vi "CameraSetup.vi"() -> ()   [LabVIEW 2015, in "CameraSetup.lvlib"]
uses:
  CameraSetup.lvlib
  <vilib>/userdefined/High Color/IMAQdx.ctl
  <vilib>/vision/driver/IMAQdx.llb/IMAQdx Acquisition Mode.ctl
  <vilib>/vision/driver/IMAQdx.llb/IMAQdx Buffer Number Mode.ctl
  <vilib>/vision/driver/NI_Vision_Acquisition_Software.lvlib
panel:
  in  "SaveConfig":bool caption="Save"
  in  "PageTab":T1(tab)
  in  "U32":u32(slide) min=720 max=720 step=1 scale=648.0..720.0
  in  "DBL":dbl(slide)=1e-06 min=0.0 max=3.999 step=1.0 scale=0.0..3.999
  in  "String":string
  in  "Ring":u32(ring) caption="Enum" items=["Bilinear", "VNG"]
  in  "Boolean":bool
  in  "Command":bool
  in  "Grab":bool
  out "Tooltip":string
  out "Image":T2(plugin-control)
  in  "Attribute":string(tree)
  in  "Cameras List":T3
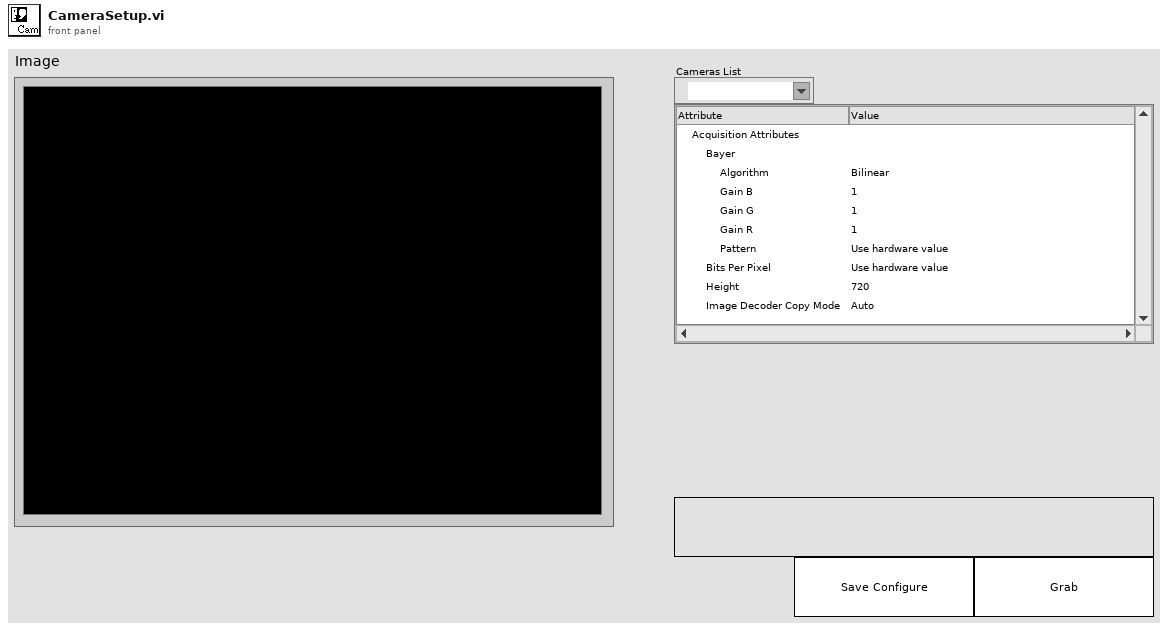
[diagram p1: front panel]
types:
  T1 = enum32{"U32", "DBL", "String", "Enum", "Bool", "Command"}
  T2 = typedef "IMAQ Image.ctl" = refnum<image>
  T3 = typedef "IMAQdx.ctl" = refnum<k21>
  T4 = cluster{"PageTab":refnum<vi>, "U32":refnum<vi>, "DBL":refnum<vi>, "String":refnum<vi>, "Enum":refnum<vi>, "Boolean":refnum<vi>, "Command":refnum<vi>}
  T5 = typedef "NI_Vision_Acquisition_Software.lvlib/IMAQdx Acquisition Mode.ctl" = enum32{"One Shot", "Continuous"}
  T6 = typedef "NI_Vision_Acquisition_Software.lvlib/IMAQdx Buffer Number Mode.ctl" = enum32{"Next", "Last", "Buffer Number", "Every", "Last New"}
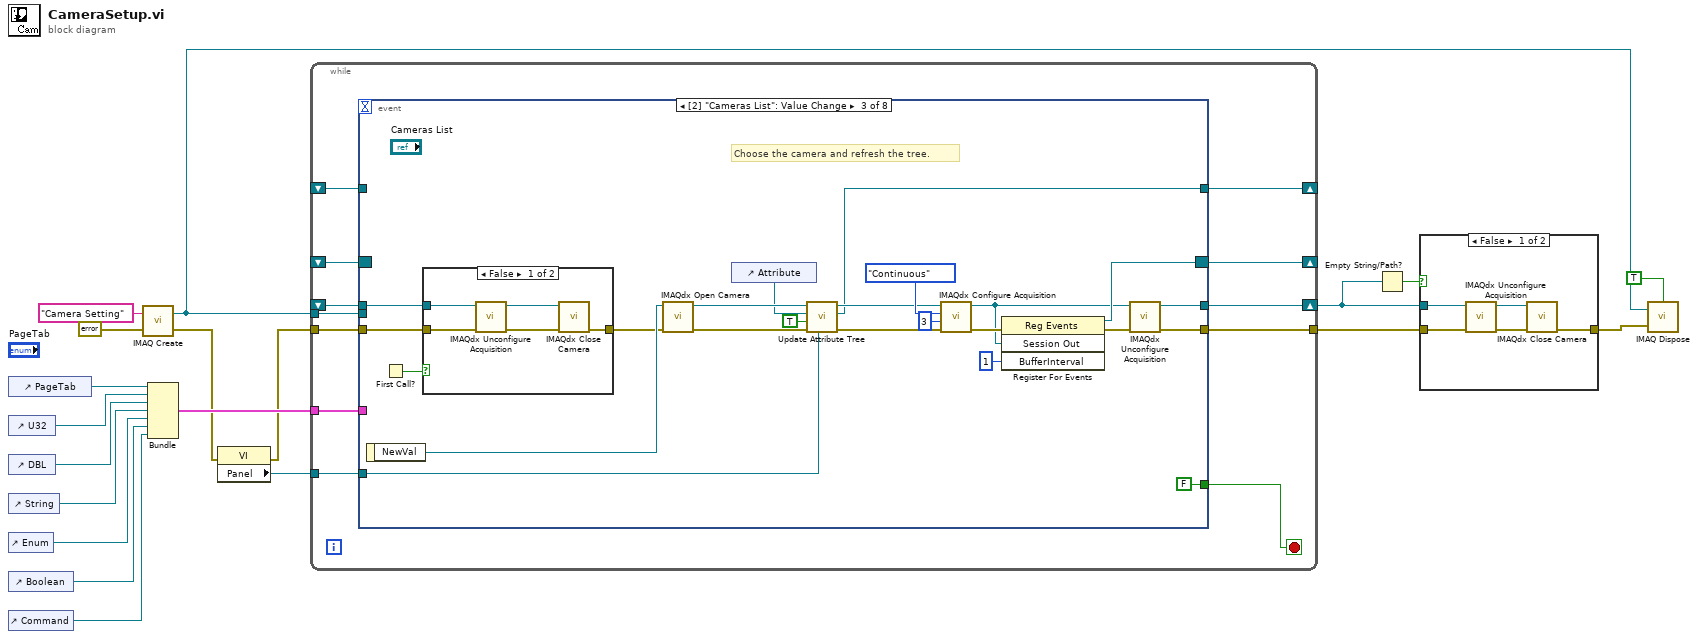
[diagram p0: block diagram]
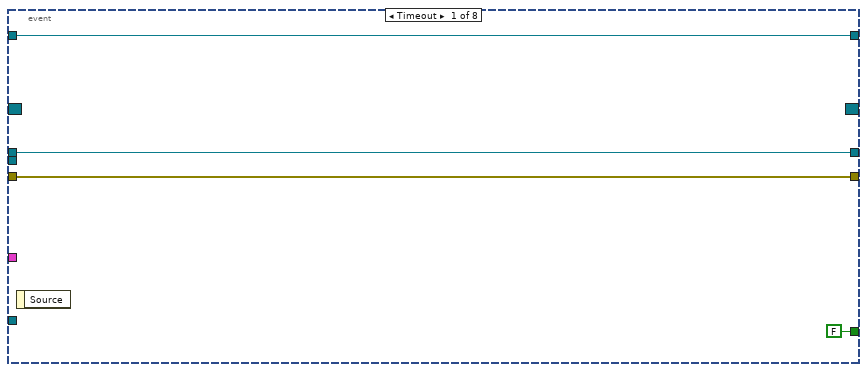
[diagram p3: hidden frame]
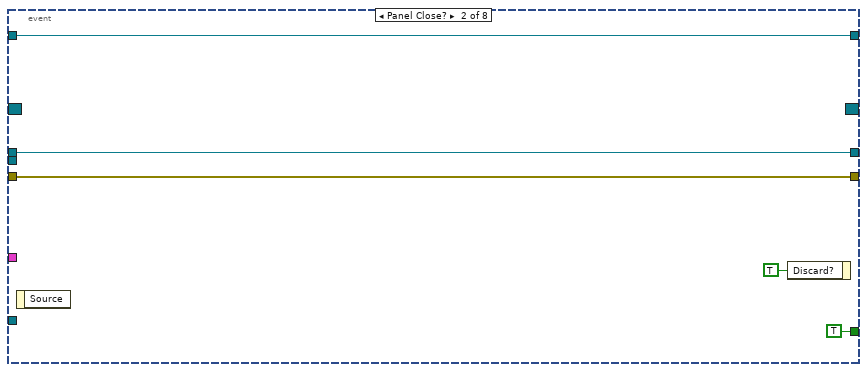
[diagram p4: hidden frame]
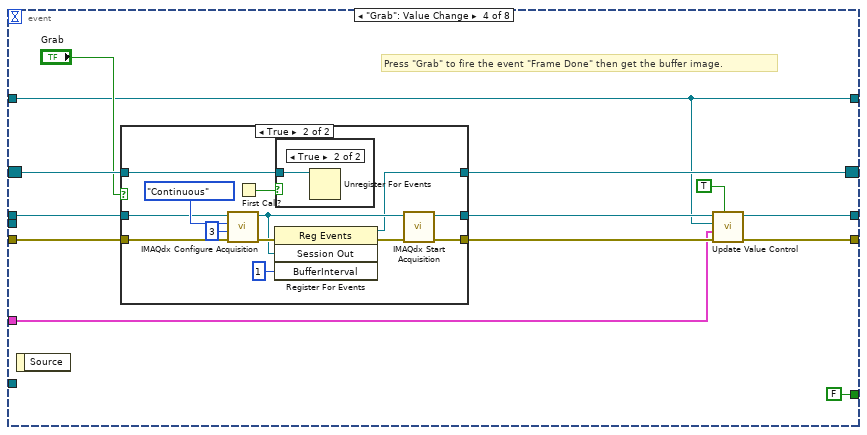
[diagram p6: hidden frame]
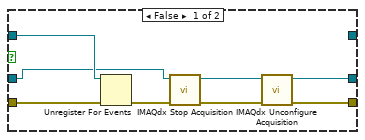
[diagram p7: hidden frame]
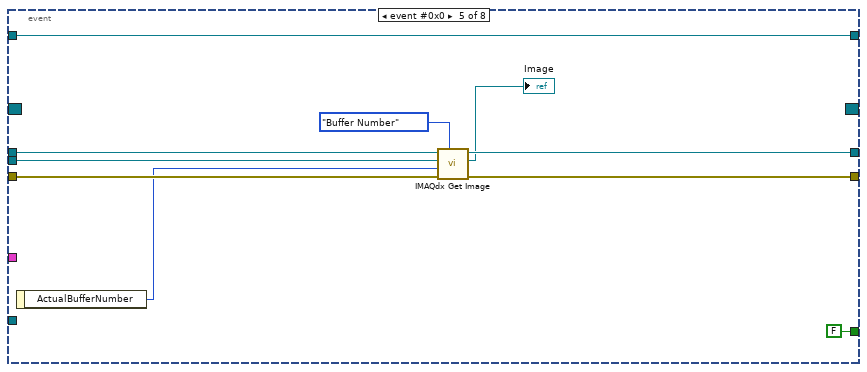
[diagram p9: hidden frame]
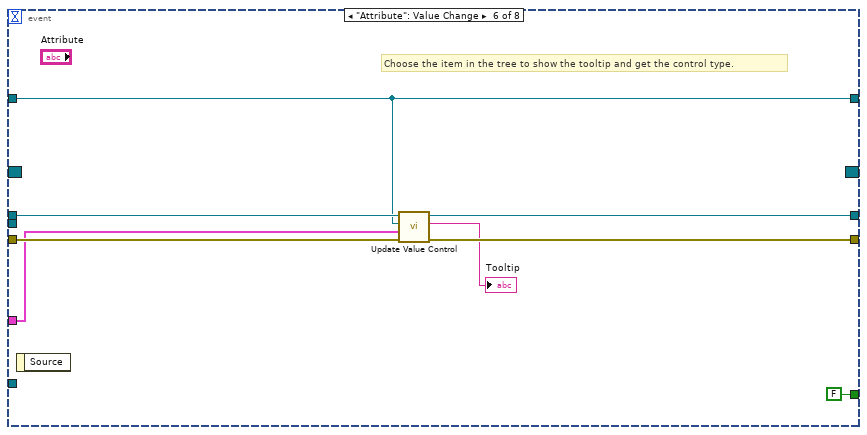
[diagram p10: hidden frame]
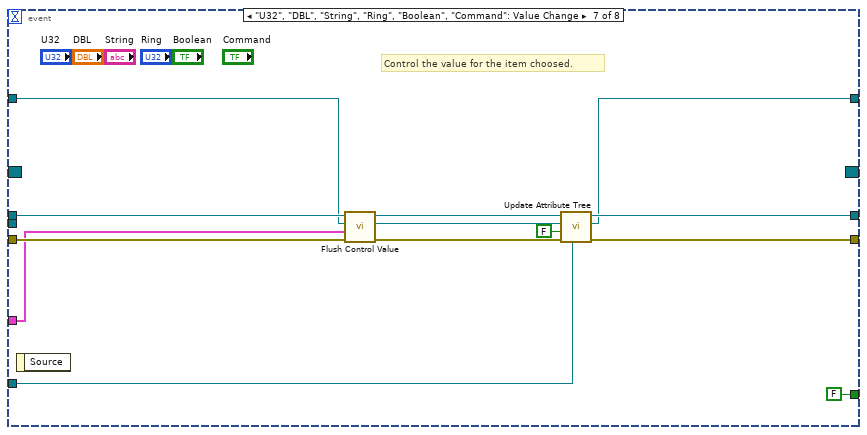
[diagram p11: hidden frame]
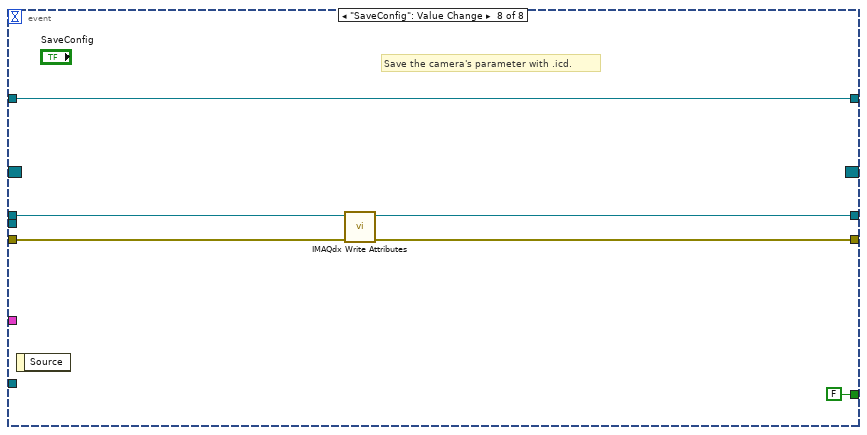
[diagram p12: hidden frame]
diagram:
  n1 = control-ref of="PageTab"() -> (w8:refnum<vi>)
  n2 = control-ref of="U32"() -> (w14:refnum<vi>)
  n3 = control-ref of="DBL"() -> (w13:refnum<vi>)
  n4 = control-ref of="String"() -> (w11:refnum<vi>)
  n5 = control-ref of="Enum"() -> (w10:refnum<vi>)
  n6 = control-ref of="Boolean"() -> (w9:refnum<vi>)
  n7 = control-ref of="Command"() -> (w12:refnum<vi>)
  n8 = call "IMAQ Create"("Image Name"="Camera Setting", "error in (no error)"=errorcluster {"status"=FALSE, "code"=0, "source"=""} ("error constant")) -> ("New Image"=w15:T2, "error out"=w6:errorcluster)  [unwired: 3 in]
  n9 = Bundle("PageTab"=w8, "U32"=w14, "DBL"=w13, "String"=w11, "Enum"=w10, "Boolean"=w9, "Command"=w12) -> (w7:T4)  [unwired: 1 in]
  n10 = property class="VI"(error in=w6) -> (error out=w5:errorcluster, "Panel"=w4:refnum<vi>)  [unwired: 1 in, 1 out]
  n11 = while {
    shift-right: [w31] -> _
    shift-left: _ -> [w30]
    shift-right: [w29] -> w1
    shift-left: _ -> [w28]
    tunnel: w15 -> [w26]
    shift-right: [w24] -> _
    shift-left: _ -> [w23]
    tunnel: w7 -> [w22]
    tunnel: w4 -> [w21]
    tunnel: w5 -> [w27]
    tunnel: [w25] -> w17
    stop <- w20 stop-if-true
    n12 = event shown="[2] \"Cameras List\": Value Change" {
      selector: w30 -> [_ _ _ w79 _ _ _ _]
      dyn-events: [_ _ w59 w74 _ _ _ _] -> w31
      timeout: _ -> [_ _ _ _ _ _ _ _]
      tunnel: [FALSE TRUE FALSE FALSE FALSE FALSE FALSE FALSE] -> w20
      tunnel: [w35 w37 w56 w81 w108 w120 w131 w139] -> w29
      tunnel: [w34 w40 w55 w82 w113 w119 w130 w140] -> w25
      tunnel: w28 -> [w35 w37 w52 w77 w111 w121 w135 w138]
      tunnel: w27 -> [w34 w40 w51 w78 w114 w122 w134 w141]
      tunnel: w26 -> [_ _ _ _ w109 _ _ _]
      tunnel: [w33 w36 w44 w71 w106 w116 w127 w137] -> w24
      tunnel: w23 -> [w33 w36 _ w71 w106 w116 w129 w137]
      tunnel: w22 -> [_ _ _ w70 _ w117 w126 _]
      tunnel: w21 -> [_ _ w42 _ _ _ w125 _]
      event Timeout {
        n13 = event-data() -> ()  [unwired: 1 in, 1 out]
      }
      event Panel Close? {
        n14 = event-data() -> ()  [unwired: 1 in, 1 out]
        n15 = event-data("Discard?"=TRUE) -> ()  [unwired: 1 in, 1 out]
      }
      event Value Change {
        # "Choose the camera and refresh the tree."
        n16 = event-data() -> ("NewVal"=w54:T3)  [unwired: 1 in]
        n17 = First Call?() -> (First Call?: T/F=w53:bool)
        n18 = case shown="False" w53 {
          tunnel: w52 -> [w66 _]
          tunnel: w51 -> [w65 w69]
          tunnel: [w64 w69] -> w50
          frame False {
            n19 = call <vilib>:"IMAQdx Unconfigure Acquisition.vi"("error in"=w65, "Session In"=w66) -> ("error out"=w67:errorcluster, "Session Out"=w68:T3)  [unwired: 8 in]
            n20 = call <vilib>:"IMAQdx Close Camera.vi"("error in"=w67, "Session In"=w68) -> ("error out"=w64:errorcluster)  [unwired: 9 in]
          }
          frame True {
          }
        }
        n21 = call <vilib>:"IMAQdx Open Camera.vi"("error in"=w50, "Session In"=w54) -> ("error out"=w43:errorcluster, "Session Out"=w47:T3)  [unwired: 8 in]
        n22 = control-ref of="Attribute"() -> (w46:refnum<vi>)
        n23 = call "Update Attribute Tree.vi"("Panel Refnum In"=w42, "error in"=w43, "Flush Tree?"=TRUE, "Tree Control In"=w46, "Camera Name In"=w47) -> ("error out"=w49:errorcluster, "Tree Control Out"=w44:refnum<vi>, "Session Out"=w48:T3)  [unwired: 4 in]
        n24 = call <vilib>:"IMAQdx Configure Acquisition.vi"("error in"=w49, "Number of Buffers"=u32 3, "Continuous?"=IMAQdx_Acquisition_Mode."Continuous", "Session In"=w48) -> ("error out"=w61:errorcluster, "Session Out"=w57:T3)  [unwired: 6 in]
        n25 = register-events(error in=w61, w57, u32 1 ("BufferInterval")) -> (reference out=w59:refnum<event-registration>, error out=w58:errorcluster)  [unwired: 1 in]
        n26 = call <vilib>:"IMAQdx Unconfigure Acquisition.vi"("error in"=w58, "Session In"=w57) -> ("error out"=w55:errorcluster, "Session Out"=w56:T3)  [unwired: 8 in]
      }
      event "Grab": Value Change {
        # "Press \"Grab\" to fire the event \"Frame Done\" then get the buffer image."
        n27 = event-data() -> ()  [unwired: 1 in, 1 out]
        n28 = case shown="True" "Grab" {
          tunnel: [w87 w94] -> w80
          tunnel: w79 -> [w86 w98]
          tunnel: w78 -> [w90 w97]
          tunnel: w77 -> [w85 w96]
          tunnel: [w83 w95] -> w76
          tunnel: [_ w91] -> w74
          frame False {
            n29 = Unregister For Events(event registration refnum=w86, error in=w90) -> (error out=w89:errorcluster)
            n30 = call <vilib>:"IMAQdx Stop Acquisition.vi"("error in"=w89, "Session In"=w85) -> ("error out"=w88:errorcluster, "Session Out"=w84:T3)  [unwired: 8 in]
            n31 = call <vilib>:"IMAQdx Unconfigure Acquisition.vi"("error in"=w88, "Session In"=w84) -> ("error out"=w87:errorcluster, "Session Out"=w83:T3)  [unwired: 8 in]
          }
          frame True {
            n32 = call <vilib>:"IMAQdx Configure Acquisition.vi"("error in"=w97, "Number of Buffers"=u32 3, "Continuous?"=IMAQdx_Acquisition_Mode."Continuous", "Session In"=w96) -> ("error out"=w102:errorcluster, "Session Out"=w92:T3)  [unwired: 6 in]
            n33 = First Call?() -> (First Call?: T/F=w99:bool)
            n34 = register-events(error in=w102, w92, u32 1 ("BufferInterval")) -> (reference out=w91:refnum<event-registration>, error out=w93:errorcluster)  [unwired: 1 in]
            n35 = case shown="True" w99 {
              tunnel: w98 -> [_ w104]
              frame False {
              }
              frame True {
                n36 = Unregister For Events(event registration refnum=w104) -> ()  [unwired: 1 in, 1 out]
              }
            }
            n37 = call <vilib>:"IMAQdx Start Acquisition.vi"("error in"=w93, "Session In"=w92) -> ("error out"=w94:errorcluster, "Session Out"=w95:T3)  [unwired: 8 in]
          }
        }
        n38 = call "Update Value Control.vi"("Force update?"=TRUE, "error in (no error)"=w80, "Tab Control Ref In"=w70, "Tree Control In"=w71, "Session In"=w76) -> ("error out"=w82:errorcluster, "Session Out"=w81:T3)  [unwired: 3 in, 2 out]
      }
      event event #0x0 {
        n39 = event-data() -> ("ActualBufferNumber"=w110:u32)  [unwired: 1 in]
        n40 = call <vilib>:"IMAQdx Get Image.vi"("Buffer Number Mode (Next)"=IMAQdx_Buffer_Number_Mode."Buffer Number", "error in"=w114, "Buffer Number In"=w110, "Image In"=w109, "Session In"=w111) -> ("error out"=w113:errorcluster, "Image Out"=→"Image":T2, "Session Out"=w108:T3)  [unwired: 3 in, 1 out]
      }
      event "Attribute": Value Change {
        # "Choose the item in the tree to show the tooltip and get the control type."
        n41 = event-data() -> ()  [unwired: 1 in, 1 out]
        n42 = call "Update Value Control.vi"("error in (no error)"=w122, "Tab Control Ref In"=w117, "Tree Control In"=w116, "Session In"=w121) -> ("error out"=w119:errorcluster, "Tooltip"=→"Tooltip":string, "Session Out"=w120:T3)  [unwired: 4 in, 1 out]
      }
      event "U32", "DBL", "String", "Ring", "Boolean", "Command": Value Change {
        # "Control the value for the item choosed."
        n43 = event-data() -> ()  [unwired: 1 in, 1 out]
        n44 = call "Flush Control Value.vi"("error in (no error)"=w134, "Tab Control Ref In"=w126, "Tree Control In"=w129, "Session In"=w135) -> ("error out"=w132:errorcluster, "Tree Control Out"=w128:refnum<vi>, "Session Out"=w133:T3)  [unwired: 5 in]
        n45 = call "Update Attribute Tree.vi"("Panel Refnum In"=w125, "error in"=w132, "Flush Tree?"=FALSE, "Tree Control In"=w128, "Camera Name In"=w133) -> ("error out"=w130:errorcluster, "Tree Control Out"=w127:refnum<vi>, "Session Out"=w131:T3)  [unwired: 4 in]
      }
      event "SaveConfig": Value Change {
        # "Save the camera's parameter with .icd."
        n46 = event-data() -> ()  [unwired: 1 in, 1 out]
        n47 = call <vilib>:"IMAQdx Write Attributes.vi"("error in"=w141, "Session In"=w138) -> ("error out"=w140:errorcluster, "Session Out"=w139:T3)  [unwired: 8 in]
      }
    }
  }
  n48 = Empty String/Path?(string/path=w1) -> (empty?=w2:bool)
  n49 = case shown="False" w2 {
    tunnel: w17 -> [w146 w147]
    tunnel: [w143 w147] -> w16
    tunnel: w1 -> [w142 _]
    frame False {
      n50 = call <vilib>:"IMAQdx Unconfigure Acquisition.vi"("error in"=w146, "Session In"=w142) -> ("error out"=w145:errorcluster, "Session Out"=w144:T3)  [unwired: 8 in]
      n51 = call <vilib>:"IMAQdx Close Camera.vi"("error in"=w145, "Session In"=w144) -> ("error out"=w143:errorcluster)  [unwired: 9 in]
    }
    frame True {
    }
  }
  n52 = call "IMAQ Dispose"("All Images? (No)"=TRUE, "Image"=w15, "error in (no error)"=w16) -> ()  [unwired: 3 in, 1 out]
